vi "ma_SML Linear Weighting (complex input).vi"(3 "reset?":bool, 4 "settings":T1, 5 "x":cdb[](array[numeric]) format="%.2f") -> (0 "data ready?":bool, 1 "averaged sofar":dbl format="%.2f", 2 "y":cdb[](array[numeric]) format="%.2f")   [LabVIEW 2020, in "NI_MAPro.lvlib"]
uses:
  NI_MAPro.lvlib
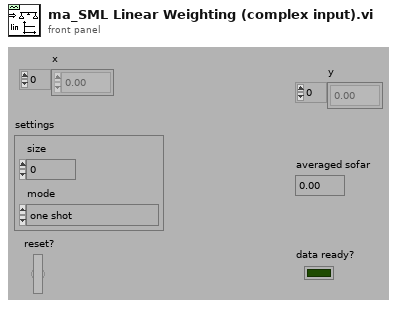
[diagram p1: front panel]
types:
  T1 = cluster{"size":dbl, "mode":enum16{"one shot", "auto restart one shot", "moving average", "continuous"}}
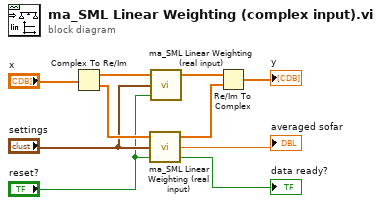
[diagram p0: block diagram]
diagram:
  n1 = Complex To Re/Im(x + iy="x") -> (x=w10:dbl[], y=w9:dbl[])
  n2 = call "ma_SML Linear Weighting (real input).vi"("reset?"="reset?", "settings"="settings", "x"=w9) -> ("data ready?"=→"data ready?":bool, "averaged sofar"=→"averaged sofar":dbl, "y"=w5:dbl[])
  n3 = call "ma_SML Linear Weighting (real input).vi"("reset?"="reset?", "settings"="settings", "x"=w10) -> ("y"=w6:dbl[])  [unwired: 2 out]
  n4 = Re/Im To Complex(1:w5, 2:w6) -> (0:→"y":cdb[])
